vi "Superdense Coding.vi"() -> ()   [LabVIEW 2020]
uses:
  QuSim/QuVI_Wire (initial).vi
  QuSim/QuVI_Wire (added).vi
  Gates/Polymorphs/vControl_e.vi
  Gates/Polymorphs/Pauli-X_t.vi
  Gates/Polymorphs/Pauli-Z_s.vi
  Gates/Polymorphs/Pauli-X_s.vi
panel:
  out "Classical bit 2":bool
  out "Classical bit 1":bool
  in  "Classical bit 1":bool
  in  "Classical bit 2":bool=TRUE
  # "Superdense Coding Example"
  # "*Open the block diagram for the circuit view (Ctrl+E)"
  # "Demonstrates transmitting 2 classical bits using a single qubit and entanglement.\n\nAlice encodes a 2-bit message (00, 01, 10, 11) onto one half of an entangled pair using logic gates (I, X, Z, ZX). Bob receives the qubit and performs a Bell measurement to recover the two classical bits. This example highlights how entanglement allows for information density beyond classical limits."
  # "Alice"
  # "Bob"
  # "Alice  sends a 2-bit message (00, 01, 10, or 11) to Bob.\n\nUse the switches 'Classical bit 1' and 'Classical bit 2' to select your message."
  # "Bob receives Alice's qubit and decodes it.\nThe LEDs show the message Bob recovered.\n\nNotice: Bob recovers TWO bits of information, even though Alice only sent ONE qubit!"
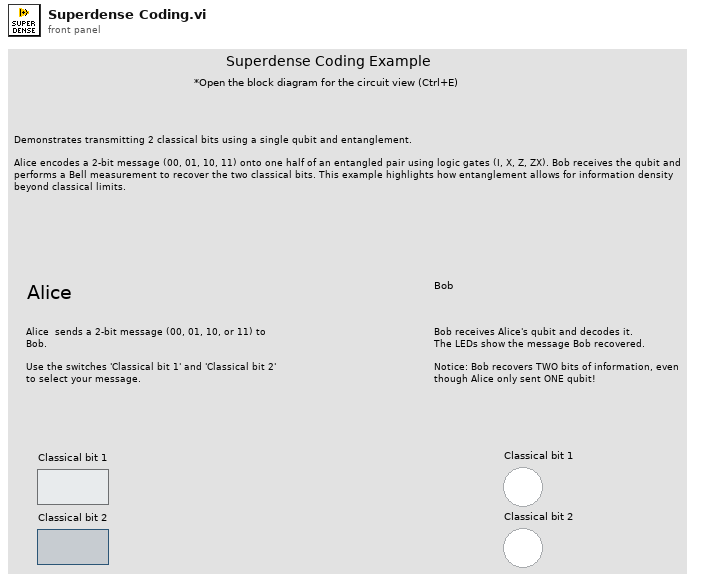
[diagram p1: front panel]
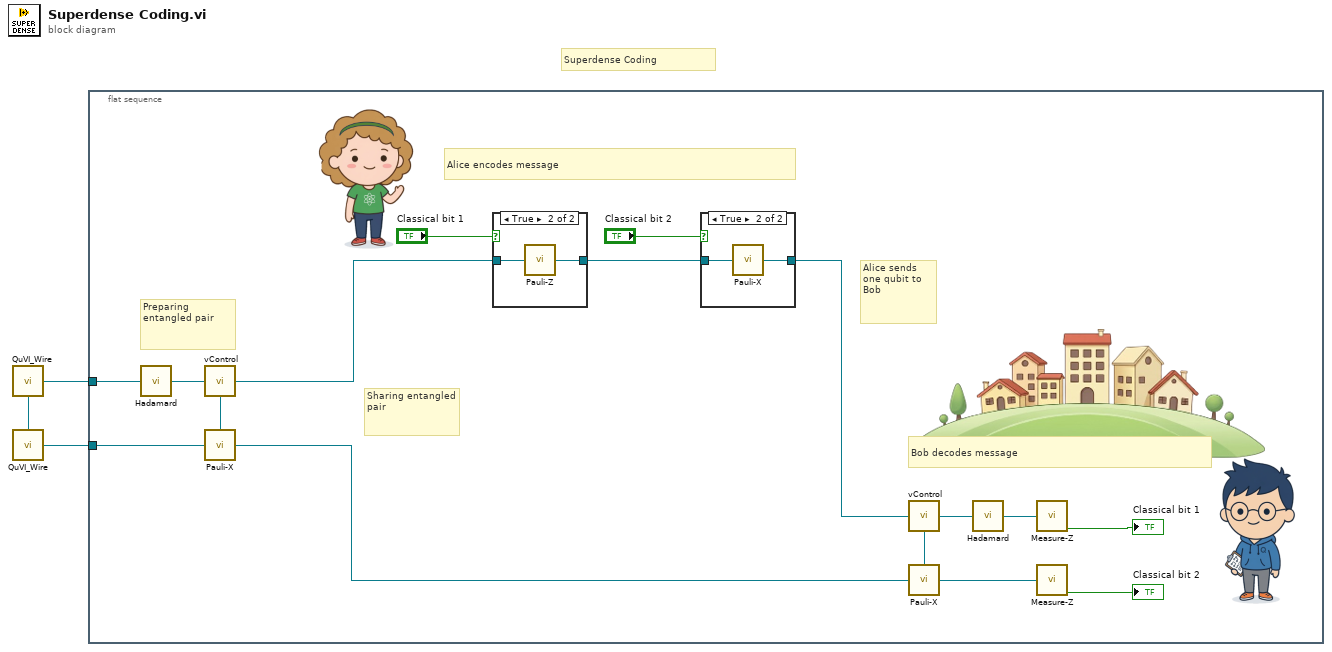
[diagram p0: block diagram]
diagram:
  # "Superdense Coding"
  n1 = call-poly "QuVI_Wire.vi"() -> ("QuWire out"=w3:refnum<class "QuWire.lvclass">, "Stack out"=w2:refnum<class "QuSim.lvclass">)  [unwired: 14 in]
  n2 = call-poly "QuVI_Wire.vi"("Stack in"=w2) -> ("QuWire out"=w1:refnum<class "QuWire.lvclass">)  [unwired: 13 in, 1 out]
  n3 = flat-sequence {
    tunnel: w3 -> [w19]
    tunnel: w1 -> [w16]
    frame #0 {
      # "Preparing entangled pair"
      # "Sharing entangled pair"
      # "Alice sends one qubit to Bob"
      # "Bob decodes message"
      # "Alice encodes message"
      n4 = call "Hadamard.vi"("QuWire in"=w19) -> ("QuWire out"=w17:refnum<class "QuWire.lvclass">)  [unwired: 14 in]
      n5 = call-poly "vControl.vi"("QuWire in"=w17) -> ("QuWire out"=w12:refnum<class "QuWire.lvclass">, "v Ctrl out"=w18:refnum<class "CtrlLine.lvclass">)  [unwired: 13 in]
      n6 = call-poly "Pauli-X.vi"("v Ctrl  in"=w18, "QuWire in"=w16) -> ("QuWire out"=w9:refnum<class "QuWire.lvclass">)  [unwired: 13 in]
      n7 = case shown="True" "Classical bit 1" {
        tunnel: w12 -> [w20 w22]
        tunnel: [w20 w21] -> w13
        frame False {
        }
        frame True {
          n8 = call-poly "Pauli-Z.vi"("QuWire in"=w22) -> ("QuWire out"=w21:refnum<class "QuWire.lvclass">)  [unwired: 14 in]
        }
      }
      n9 = case shown="True" "Classical bit 2" {
        tunnel: w13 -> [w23 w25]
        tunnel: [w23 w24] -> w10
        frame False {
        }
        frame True {
          n10 = call-poly "Pauli-X.vi"("QuWire in"=w25) -> ("QuWire out"=w24:refnum<class "QuWire.lvclass">)  [unwired: 14 in]
        }
      }
      n11 = call-poly "vControl.vi"("QuWire in"=w10) -> ("QuWire out"=w8:refnum<class "QuWire.lvclass">, "v Ctrl out"=w11:refnum<class "CtrlLine.lvclass">)  [unwired: 13 in]
      n12 = call-poly "Pauli-X.vi"("v Ctrl  in"=w11, "QuWire in"=w9) -> ("QuWire out"=w6:refnum<class "QuWire.lvclass">)  [unwired: 13 in]
      n13 = call "Hadamard.vi"("QuWire in"=w8) -> ("QuWire out"=w7:refnum<class "QuWire.lvclass">)  [unwired: 14 in]
      n14 = call "Measure-Z.vi"("QuWire in"=w7) -> ("Classical bit"=→"Classical bit 1":bool)  [unwired: 13 in, 1 out]
      n15 = call "Measure-Z.vi"("QuWire in"=w6) -> ("Classical bit"=→"Classical bit 2":bool)  [unwired: 13 in, 1 out]
    }
  }
